vi "DataStorageDataSetPacketRoutedMessage_Create.vi"(7 "Header":T3, 8 "error in (no error)":errorcluster, 9 "DataSet":T1, 10 "IRoutingSource":T2) -> (0 "error out":errorcluster, 3 "Message":T5)   [LabVIEW 2017]
uses:
  <vilib>/addons/InsightCM/MessageBus/Base/controls/Message.ctl
  <vilib>/addons/InsightCM/MessageBus/Base/controls/MessageHeader.ctl
  <vilib>/addons/InsightCM/MessageBus/Base/controls/KeyValuePair.ctl
  <vilib>/addons/InsightCM/MessageBus/Base/controls/IRoutingSource.ctl
  <vilib>/addons/InsightCM/MessageBus/Base/controls/DataSetPacket.ctl
  <vilib>/addons/InsightCM/MessageBus/Base/controls/MessageClassType.ctl
  <vilib>/addons/InsightCM/Utilities/PropertyHelpers/PropertyHelpers.lvlib
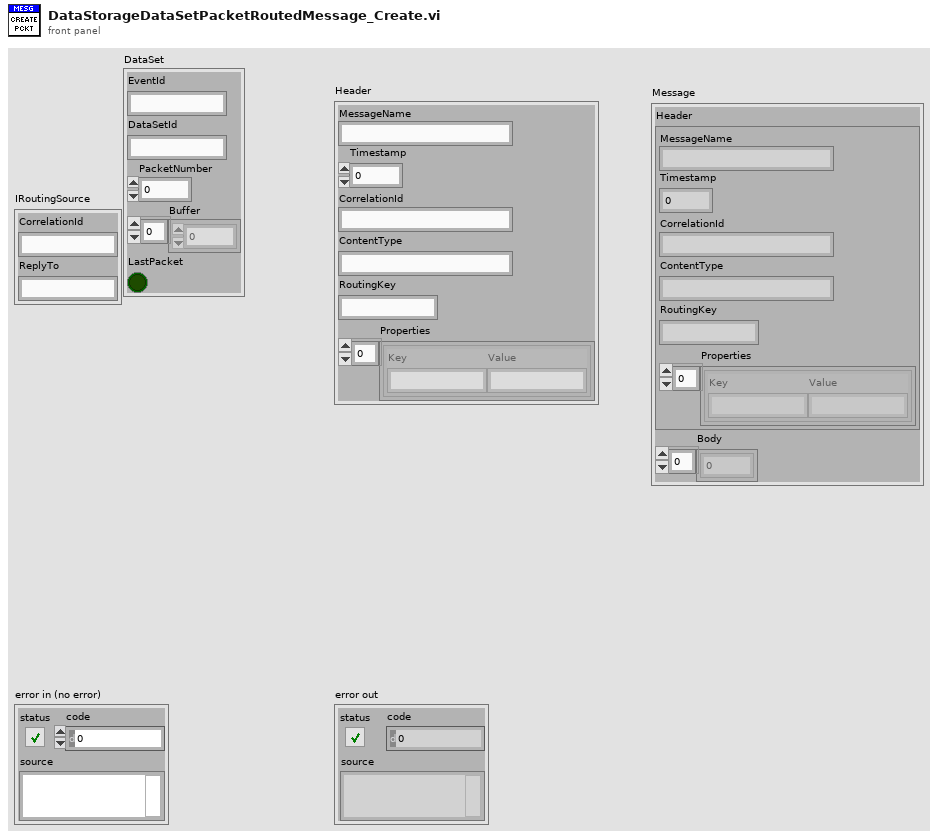
[diagram p1: front panel]
types:
  T1 = typedef "DataSetPacket.ctl" = cluster{"EventId":string, "DataSetId":string, "PacketNumber":i32, "Buffer":u8[], "LastPacket":bool}
  T2 = typedef "IRoutingSource.ctl" = cluster{"CorrelationId":string, "ReplyTo":string}
  T3 = typedef "MessageHeader.ctl" = cluster{"MessageName":string, "Timestamp":i64, "CorrelationId":string, "ContentType":string, "RoutingKey":string, "Properties":T4[]}
  T4 = typedef "KeyValuePair.ctl" = cluster{"Key":string, "Value":string}
  T5 = typedef "Message.ctl" = cluster{"Header":T3, "Body":u8[]}
  T6 = typedef "MessageClassType.ctl" = enum16{"Request", "Response", "Broadcast", "RoutedMessage"}
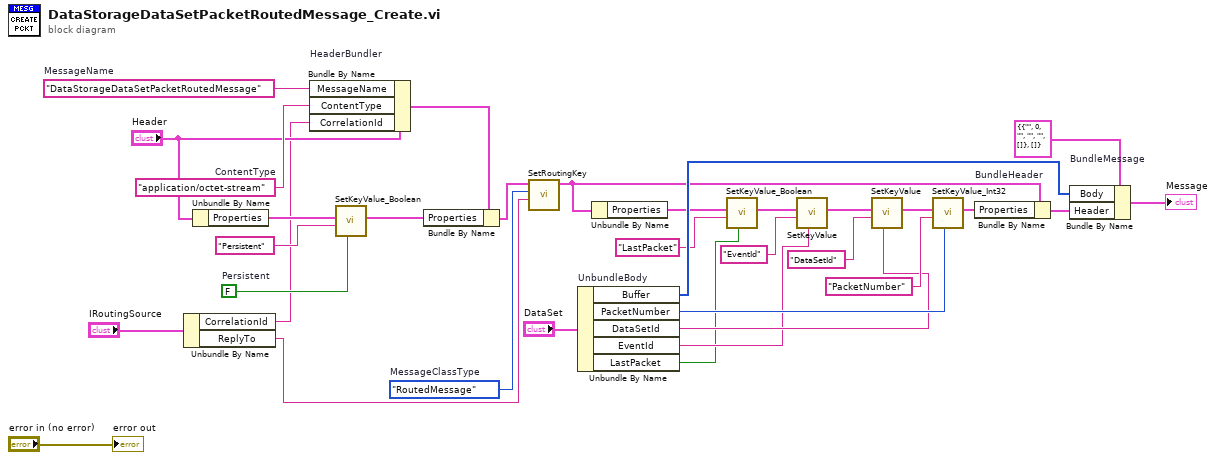
[diagram p0: block diagram]
diagram:
  w29 = MessageClassType."RoutedMessage"  # MessageClassType
  w24 = FALSE  # Persistent
  w30 = "DataStorageDataSetPacketRoutedMessage"  # MessageName
  w27 = "application/octet-stream"  # ContentType
  n1 = Unbundle By Name("IRoutingSource") -> ("CorrelationId"=w16:string, "ReplyTo"=w15:string)
  n2 = Unbundle By Name("Header") -> ("Properties"=w26:T4[])
  n3 = Bundle By Name "HeaderBundler"(cluster="Header", "MessageName"=w30, "ContentType"=w27, "CorrelationId"=w16) -> (w21:T3)
  n4 = call <vilib>:"SetKeyValue_Boolean.vi"("value"=w24, "key"="Persistent" ("Key"), "key value pairs"=w26) -> ("key value pairs out"=w20:T4[])  [unwired: 8 in]
  n5 = Bundle By Name(cluster=w21, "Properties"=w20) -> (w22:T3)
  n6 = call <vilib>:"SetRoutingKey.vi"("SendTo"=w15, "MessageClassType"=w29, "Message Header in"=w22) -> ("Message Header out"=w23:T3)  [unwired: 8 in]
  n7 = Unbundle By Name "UnbundleBody"("DataSet") -> ("Buffer"=w32:u8[], "PacketNumber"=w11:i32, "DataSetId"=w10:string, "EventId"=w5:string, "LastPacket"=w1:bool)
  n8 = Unbundle By Name(w23) -> ("Properties"=w4:T4[])
  n9 = call <vilib>:"SetKeyValue_Boolean.vi"("value"=w1, "key"="LastPacket" ("Key"), "key value pairs"=w4) -> ("key value pairs out"=w3:T4[])  [unwired: 8 in]
  n10 = call <vilib>:"SetKeyValue.vi"("value"=w5, "key"="EventId" ("Key"), "key value pairs"=w3) -> ("key value pairs out"=w7:T4[])  [unwired: 8 in]
  n11 = call <vilib>:"SetKeyValue.vi"("value"=w10, "key"="DataSetId" ("Key"), "key value pairs"=w7) -> ("key value pairs out"=w14:T4[])  [unwired: 8 in]
  n12 = call <vilib>:"SetKeyValue_Int32.vi"("value"=w11, "key"="PacketNumber" ("Key"), "key value pairs"=w14) -> ("key value pairs out"=w13:T4[])  [unwired: 8 in]
  n13 = Bundle By Name "BundleHeader"(cluster=w23, "Properties"=w13) -> (w31:T3)
  n14 = Bundle By Name "BundleMessage"(cluster=T5 {"Header"={"MessageName"="", "Timestamp"=0, "CorrelationId"="", "ContentType"="", "RoutingKey"="", "Properties"=[]}, "Body"=[]} ("Message"), "Body"=w32, "Header"=w31) -> (→"Message":T5)
  "error out" <- "error in (no error)"
